vi "FV-Running_average_complex.vi"(7 "# AVG":i32=100, 10 "in":cdb[](array[numeric])) -> (2 "Out":cdb[](array[numeric]))   [LabVIEW 2020, in "FV-file_viewer.lvlib"]
uses:
  FV-file_viewer.lvlib
panel:
  out "s? t:f":i32
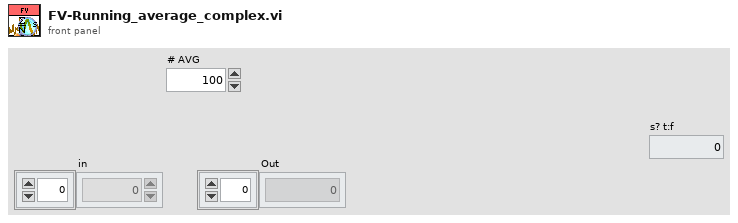
[diagram p1: front panel]
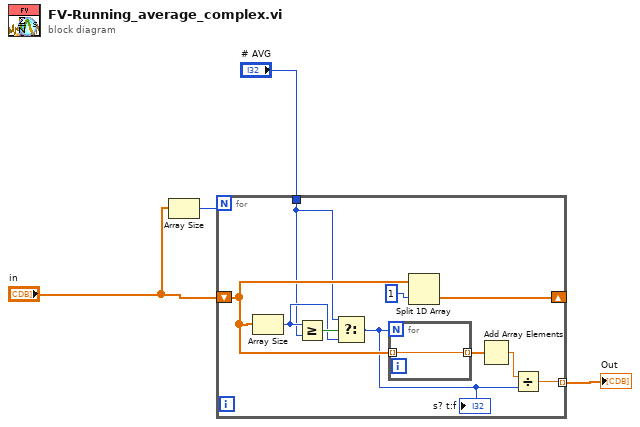
[diagram p0: block diagram]
diagram:
  n1 = Array Size(array="in") -> (size(s)=w4:i32)
  n2 = for {
    N: w4 -> [_]
    shift-right: [w13] -> _
    shift-left: "in" -> [w9]
    tunnel: [w10] -> w2 mode=indexing
    tunnel: "# AVG" -> [w5]
    n3 = Array Size(array=w9) -> (size(s)=w7:i32)
    n4 = Greater Or Equal?(x=w7, y=w5) -> (x >= y?=w8:bool)
    n5 = Select(t=w5, s=w8, f=w7) -> (s? t:f=w6:i32)
    "s? t:f" <- w6
    n6 = for {
      N: w6 -> [_]
      tunnel: w9 -> [w15] mode=indexing
      tunnel: [w15] -> w12 mode=indexing
    }
    n7 = Split 1D Array(array=w9, index=1) -> (second subarray=w13:cdb[])  [unwired: 1 out]
    n8 = Add Array Elements(numeric array=w12) -> (sum=w11:cdb)
    n9 = Divide(x=w11, y=w6) -> (x/y=w10:cdb)
  }
  "Out" <- w2
